vi "Do Main Action.vi"(8 "error in (no error)":errorcluster, 10 "AbstractData":refnum<class "AbstractData.lvclass">, 11 "AbstractProcessor in":refnum<class "AbstractProcessor.lvclass">) -> (0 "error out":errorcluster, 3 "AbstractProcessor out":refnum<class "AbstractProcessor.lvclass">)   [LabVIEW 2014, in "AbstractProcessor.lvclass"]
uses:
  AbstractProcessor.lvclass
  Model/Data/AbstractData/AbstractData.lvclass
  Interfaces/Pipelined Actor/Pipelined Actor.lvclass
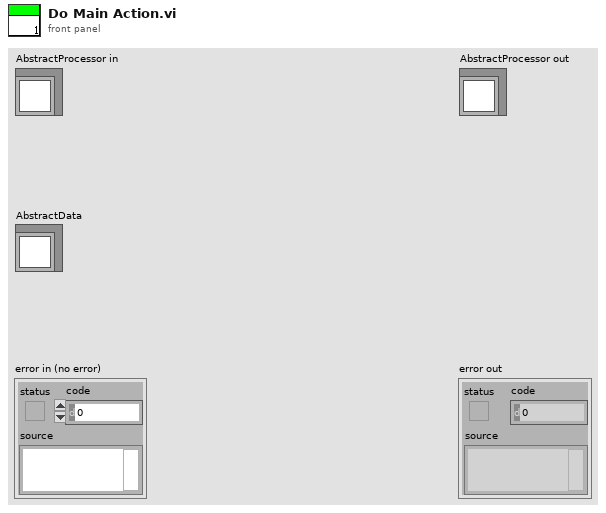
[diagram p1: front panel]
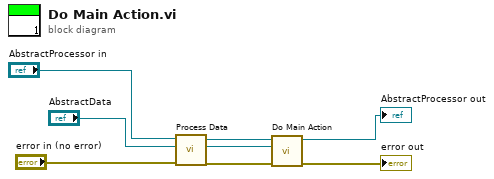
[diagram p0: block diagram]
diagram:
  n1 = call-dynamic "Process Data.vi"("error in (no error)"="error in (no error)", "AbstractData in"="AbstractData", "AbstractProcessor in"="AbstractProcessor in") -> ("error out"=w4:errorcluster, "AbstractData out"=w5:refnum<class "AbstractData.lvclass">, "AbstractProcessor out"=w6:refnum<class "AbstractProcessor.lvclass">)  [unwired: 6 in]
  n2 = call-parent "Do Main Action.vi"("error in (no error)"=w4, "AbstractData"=w5, "Pipelined Actor in"=w6) -> ("error out"=→"error out":errorcluster, "Pipelined Actor out"=→"AbstractProcessor out":refnum<class "AbstractProcessor.lvclass">)  [unwired: 7 in]
